vi "Stop.vi"(11 "Stop? (f)":bool) -> (3 "Stop":bool)   [LabVIEW 2014, in "SyncModule.lvlib"]
uses:
  SyncModule.lvlib
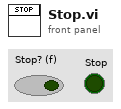
[diagram p1: front panel]
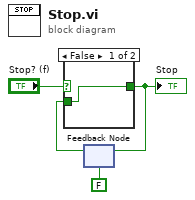
[diagram p0: block diagram]
diagram:
  n1 = feedback #1(FALSE) -> (w2:bool)
  n2 = case shown="False" "Stop? (f)" {
    selector: "Stop? (f)" -> [_ w6]
    tunnel: w2 -> [w5 _]
    tunnel: [w5 w6] -> w1
    frame False {
    }
    frame True {
    }
  }
  "Stop" <- w1
  n3 = feedback-in #1(w1) -> ()
